vi "Create Plugin Groups.vi"(8 "error in (no error)":errorcluster, 9 "String":string, 10 "dsf refnum in":T1, 11 "Section Ptr":T2 format="%.0x") -> (0 "error out":errorcluster)   [LabVIEW 2017, in "Data Sharing Framework System Explorer.lvlib"]
uses:
  Data Sharing Framework System Explorer.lvlib
  <vilib>/NI Veristand/Custom Device API/Custom Device Item Ref.ctl
  dsf core/Source/DSF Configuration API/1.0.0/Public/Controls/DSF Config Data RefNum.ctl
  dsf core/Source/DSF Configuration API/1.0.0/Public/Read Item Child IDs/Read Plugin Group IDs.vi
  dsf core/Source/DSF Configuration API/1.0.0/Public/Read Item/Read Group.vi
  <vilib>/NI Veristand/Custom Device API/Custom Device API.lvlib
  dsf core/Source/DSF Configuration API/1.0.0/DSF Configuration API.lvlib
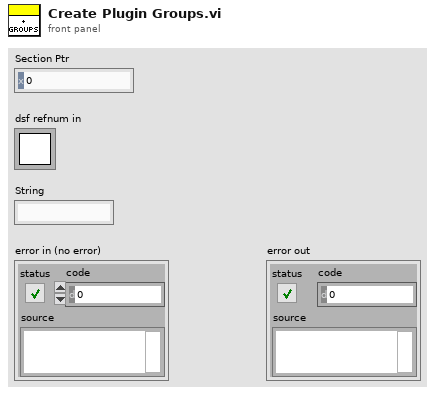
[diagram p1: front panel]
types:
  T1 = typedef "DSF Configuration API.lvlib/DSF Config Data RefNum.ctl" = refnum<k1>
  T2 = typedef "Custom Device API.lvlib/Custom Device Item Ref.ctl" = u64
  T3 = typedef "DSF Configuration API.lvlib/DSF Group Info.ctl" = cluster{"direction":T4, "timing":T5, "transfer ids":string[], "settings id":string}
  T4 = typedef "DSF Configuration API.lvlib/DSF Direction.ctl" = enum8{"Tx", "Rx"}
  T5 = typedef "DSF Configuration API.lvlib/DSF Timing Info.ctl" = cluster{"priority":i32, "decimation":i32, "offset":i32}
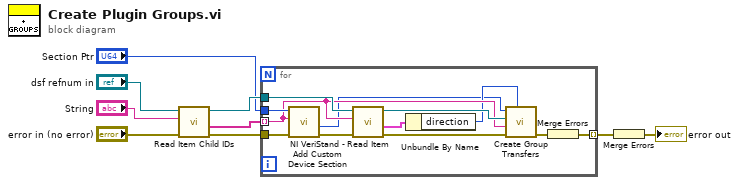
[diagram p0: block diagram]
diagram:
  n1 = call-poly "Read Item Child IDs.vi"("error in (no error)"="error in (no error)", "Plugin ID"="String", "dsf refnum"="dsf refnum in") -> ("error out"=w2:errorcluster, "Group IDs"=w1:string[], "dsf refnum out"=w8:T1)  [unwired: 5 in, 1 out]
  n2 = for {
    tunnel: w1 -> [w13] mode=indexing
    tunnel: "Section Ptr" -> [w21]
    tunnel: w2 -> [w20]
    tunnel: [w18] -> w6 mode=indexing
    tunnel: w8 -> [w16]
    n3 = call <vilib>:"NI VeriStand - Add Custom Device Section.vi"("error in (no error)"=w20, "Section Name"=w13, "Parent Ref in"=w21) -> ("error out"=w19:errorcluster, "Section Ptr"=w10:T2)  [unwired: 5 in, 2 out]
    n4 = call-poly "Read Item.vi"("error in (no error)"=w19, "Group ID"=w13, "dsf refnum"=w16) -> ("error out"=w17:errorcluster, "value"=w14:T3, "dsf refnum out"=w15:T1)  [unwired: 5 in, 1 out]
    n5 = Unbundle By Name(w14) -> ("direction"=w12:T4)
    n6 = call "Create Group Transfers.vi"("direction"=w12, "error in (no error)"=w17, "Group ID"=w13, "dsf refnum in"=w15, "Section Ptr"=w10) -> ("error out"=w11:errorcluster)  [unwired: 6 in]
    n7 = Merge Errors(w11) -> (w18:errorcluster)
  }
  n8 = Merge Errors(w6) -> (→"error out":errorcluster)
